vi "pixel_clock.vi"(10 "current iteration":u32, 11 "iterations per pixel":u32) -> ()   [LabVIEW 2010]
uses:
  <vilib>/eio/EIONode/EIONode.xnode
  <vilib>/rvi/eio/nirviEIOImplementation/nirviEIOImplementation.xnode
  <vilib>/rvi/eio/common/nirviEmuClasses.ctl
  <vilib>/rvi/eio/common/nirviEmuTemplateMethod_noerrors.vi
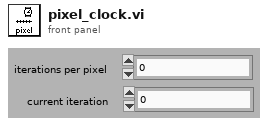
[diagram p1: front panel]
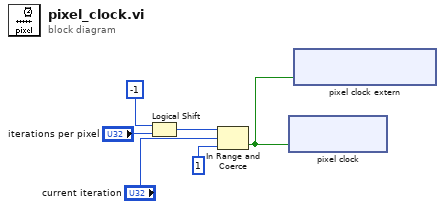
[diagram p0: block diagram]
diagram:
  n1 = Logical Shift(y=i8 -1, x="iterations per pixel") -> (x << y=w6:u32)
  n2 = In Range and Coerce(upper limit=w6, x="current iteration", lower limit=u32 1 ("upper limit")) -> (In Range?=w1:bool)  [unwired: 1 out]
  n3 = xnode "pixel clock"("pixel clock"=w1) -> ()  [unwired: 1 in, 1 out]
  n4 = xnode "pixel clock extern"("Connector1/DIO34"=w1) -> ()  [unwired: 1 in, 1 out]
